vi "ConfigCable.vi"(8 "error in (no error)":errorcluster, 10 "cable":u16(ring)=1 items=["0m", "1m", "2m"], 11 "VISA resource name":refnum<visa-resource-name>) -> (0 "error out":errorcluster, 3 "VISA resource name out":refnum<visa-resource-name>)   [LabVIEW 2016]
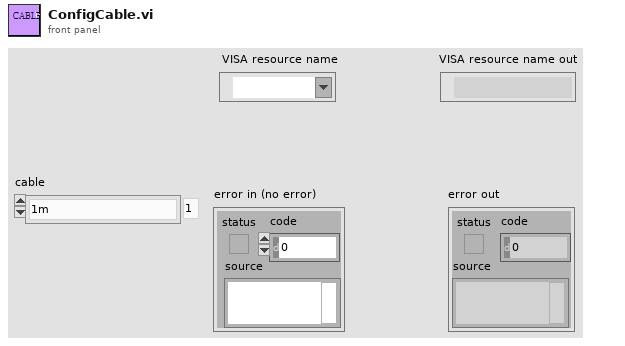
[diagram p1: front panel]
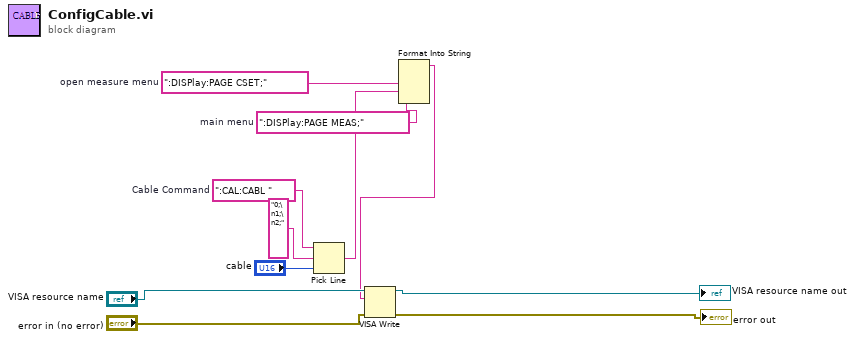
[diagram p0: block diagram]
diagram:
  w1 = ":DISPlay:PAGE MEAS;"  # main menu
  w4 = ":DISPlay:PAGE CSET;"  # open measure menu
  w9 = ":CAL:CABL "  # Cable Command
  n1 = Pick Line(string ("")=w9, multi-line string="0;\n1;\n2;", line index="cable") -> (output string=w3:string)
  n2 = Format Into String(w4, w3, w1) -> (resulting string=w2:string)  [unwired: 3 in, 1 out]
  n3 = VISA Write(VISA resource name="VISA resource name", write buffer=w2, error in (no error)="error in (no error)") -> (VISA resource name out=→"VISA resource name out":refnum<visa-resource-name>, error out=→"error out":errorcluster)  [unwired: 1 out]
